vi "IpInputFromUser.vi"(8 "IpStatus (in)":T2[](array[typedef]) {"%rtk" scale=0.0..60.0; "TimePing" scale=0.0..60.0}, 10 "IP":bool, 11 "IP STATUS(in)":T1) -> (0 "IpStatus (out)":T2[](array[typedef]) {"%rtk" scale=0.0..60.0; "TimePing" scale=0.0..60.0}, 3 "IP STATUS(out)":T1, 5 "False":bool)   [LabVIEW 2011]
uses:
  GPS String Capture Software/IP RTK status Indicator.ctl
  ArrayIpAddressesAndReportingCheckbox.ctl
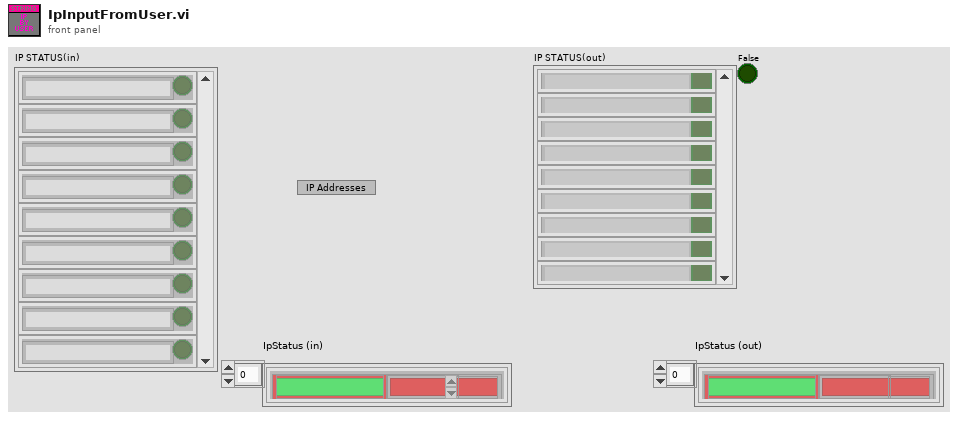
[diagram p1: front panel]
types:
  T1 = typedef "ArrayIpAddressesAndReportingCheckbox.ctl" = cluster{"IpAddress":string, "Report Errors":bool}[]
  T2 = typedef "IP RTK status Indicator.ctl" = cluster{"TimePing":dbl, "IP":string, "%rtk":dbl, "Lastrtk":string, "MinLastRTk":dbl, "RTK Count":bool[], "Last Nema Time":dbl, "Last RTK Time":dbl, "Last Ping time":dbl}
  T3 = cluster{"IpAddress":string, "Report Errors":bool}
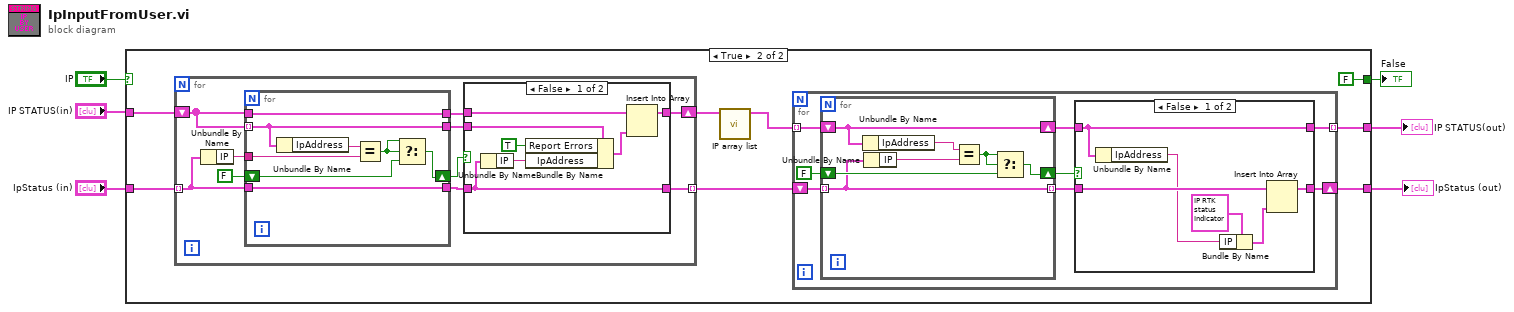
[diagram p0: block diagram]
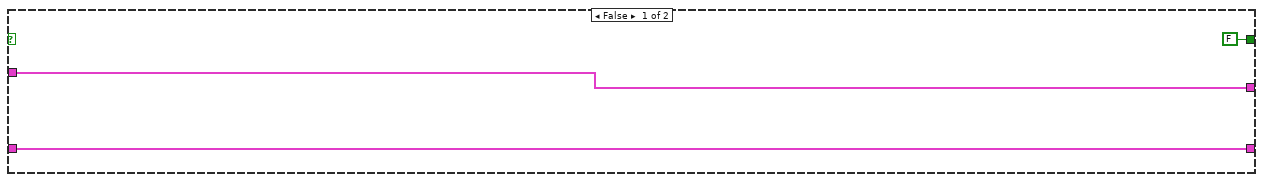
[diagram p2: hidden frame]
diagram:
  n1 = case shown="True" "IP" {
    tunnel: [w9 w17] -> w2
    tunnel: "IP STATUS(in)" -> [w9 w14]
    tunnel: "IpStatus (in)" -> [w8 w15]
    tunnel: [w8 w16] -> w4
    tunnel: [FALSE FALSE] -> w1
    frame False {
    }
    frame True {
      n2 = for {
        tunnel: w15 -> [w25] mode=indexing
        shift-right: [w22] -> w12
        shift-left: w14 -> [w19]
        tunnel: [w20] -> w13 mode=indexing
        n3 = Unbundle By Name(w25) -> ("IP"=w27:string)
        n4 = for {
          tunnel: w27 -> [w44]
          tunnel: w19 -> [w37] mode=indexing
          shift-right: [w42] -> w24
          shift-left: FALSE -> [w43]
          tunnel: w25 -> [w39]
          tunnel: [w39] -> w21
          tunnel: [w37] -> w18
          tunnel: w19 -> [w40]
          tunnel: [w40] -> w23
          n5 = Unbundle By Name(w37) -> ("IpAddress"=w38:string)
          n6 = Equal?(x=w38, y=w44) -> (x = y?=w41:bool)
          n7 = Select(t=w41, s=w41, f=w43) -> (s? t:f=w42:bool)
        }
        n8 = case shown="False" w24 {
          tunnel: w23 -> [w34 w36]
          tunnel: [w33 w36] -> w22
          tunnel: w21 -> [w32 w35]
          tunnel: [w32 w35] -> w20
          tunnel: w18 -> [w31 _]
          frame False {
            n9 = Unbundle By Name(w32) -> ("IP"=w30:string)
            n10 = Bundle By Name(cluster=w31, "Report Errors"=TRUE, "IpAddress"=w30) -> (w29:T3)
            n11 = Insert Into Array(array=w34, new element=w29) -> (w33:T1)  [unwired: 1 in]
          }
          frame True {
          }
        }
      }
      n12 = call "IP array list.vi"("IP STATUS(in)"=w12) -> ("IP STATUS(out)"=w11:T1)  [unwired: 10 in]
      n13 = for {
        tunnel: w11 -> [w51] mode=indexing
        tunnel: [w46] -> w17 mode=indexing
        shift-right: [w45] -> w16
        shift-left: w13 -> [w52]
        n14 = for {
          tunnel: w52 -> [w63] mode=indexing
          shift-right: [w64] -> w49
          shift-left: FALSE -> [w65]
          tunnel: [w63] -> w48 mode=indexing
          shift-right: [w62] -> w47
          shift-left: w51 -> [w62]
          n15 = Unbundle By Name(w62) -> ("IpAddress"=w61:string)
          n16 = Unbundle By Name(w63) -> ("IP"=w67:string)
          n17 = Equal?(x=w61, y=w67) -> (x = y?=w66:bool)
          n18 = Select(t=w66, s=w66, f=w65) -> (s? t:f=w64:bool)
        }
        n19 = case shown="False" w49 {
          tunnel: w48 -> [w57 w59]
          tunnel: w47 -> [w54 w60]
          tunnel: [w54 w60] -> w46
          tunnel: [w58 w59] -> w45
          frame False {
            n20 = Unbundle By Name(w54) -> ("IpAddress"=w53:string)
            n21 = Bundle By Name(cluster=T2 {"TimePing"=0.0, "IP"="", "%rtk"=0.0, "Lastrtk"="", "MinLastRTk"=0.0, "RTK Count"=[], "Last Nema Time"=0.0, "Last RTK Time"=0.0, "Last Ping time"=0.0} ("IP Status"), "IP"=w53) -> (w56:T2)
            n22 = Insert Into Array(array=w57, new element=w56) -> (w58:T2[])  [unwired: 1 in]
          }
          frame True {
          }
        }
      }
    }
  }
  "IpStatus (out)" <- w4
  "IP STATUS(out)" <- w2
  "False" <- w1
